vi "Get status Response.vi"(8 "error in (no error)":errorcluster, 11 "Arduino in":refnum<class "Arduino.lvclass">) -> (0 "error out":errorcluster, 2 "Response":string, 3 "Arduino out":refnum<class "Arduino.lvclass">)   [LabVIEW 2020, in "Arduino.lvclass"]
doc: "Override del papa Get Status Response"
uses:
  Arduino.lvclass
  Abstracts/Serial Device/Serial Device.lvclass
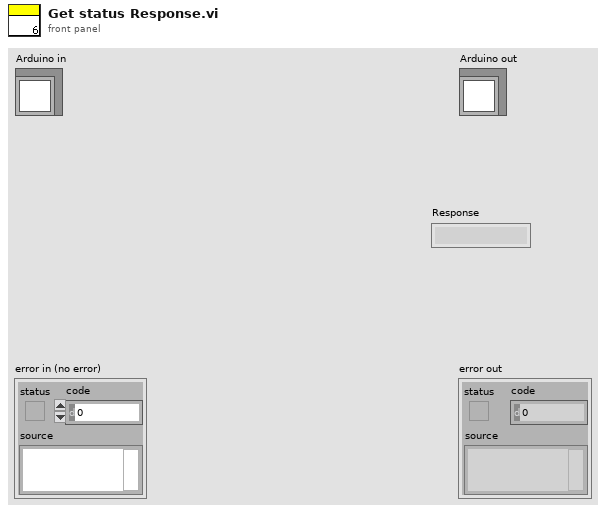
[diagram p1: front panel]
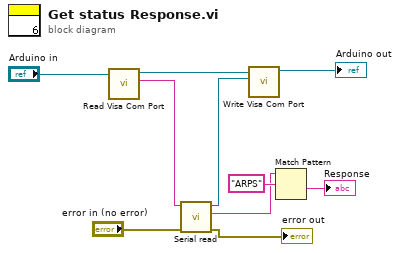
[diagram p0: block diagram]
diagram:
  n1 = call-dynamic "Read Visa Com Port.vi"("Serial Device in"="Arduino in") -> ("Visa Com Port"=w5:string, "Serial Device out"=w7:refnum<class "Arduino.lvclass">)  [unwired: 8 in, 1 out]
  n2 = call "Serial read.vi"("error in (no error)"="error in (no error)", "VISA resource name in"=w5) -> ("error out"=→"error out":errorcluster, "Respuesta"=w3:string, "VISA resource name out"=w4:refnum<visa-resource-name>)  [unwired: 7 in]
  n3 = call-dynamic "Write Visa Com Port.vi"("Visa Com Port"=w4, "Serial Device in"=w7) -> ("Serial Device out"=→"Arduino out":refnum<class "Arduino.lvclass">)  [unwired: 8 in, 1 out]
  n4 = Match Pattern(string=w3, regular expression="ARPS") -> (after substring=→"Response":string)  [unwired: 1 in, 3 out]
